vi "write_to_ini.vi"(7 "Enum":enum16{"Write", "Read variants", "Read Values"}(ring), 8 "error in (no error)":errorcluster, 9 "Input values":T1, 10 "String":string, 11 "configuration file path":path) -> (0 "error out":errorcluster, 1 "Output values":T1, 2 "section names":string[](array[string]), 3 "file path":path)   [LabVIEW 2021]
uses:
  <vilib>/Utility/config.llb/Write Key (String).vi
  <vilib>/Utility/config.llb/Read Key (String).vi
  <vilib>/Utility/config.llb/NI_LVConfig.lvlib
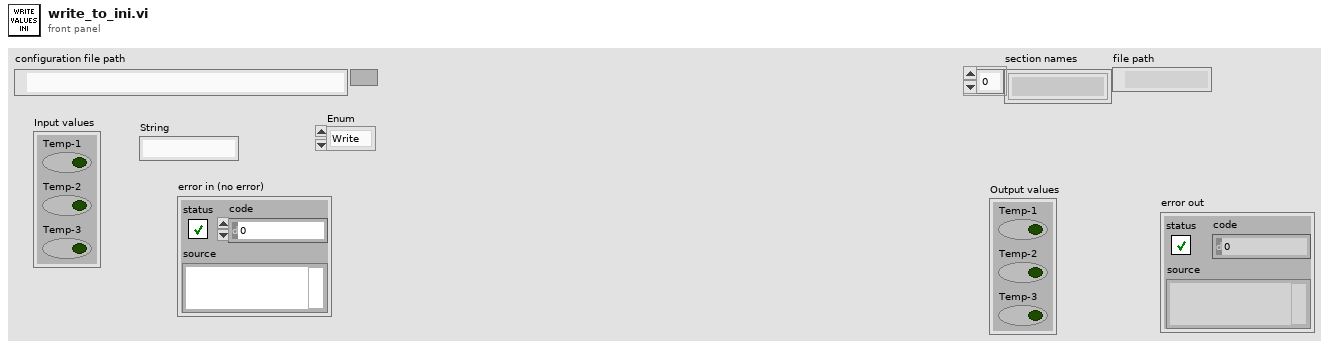
[diagram p1: front panel]
types:
  T1 = cluster{"Temp-1":bool, "Temp-2":bool, "Temp-3":bool}
  T2 = typedef "NI_LVConfig.lvlib/Config Data RefNum.ctl" = refnum<k1>
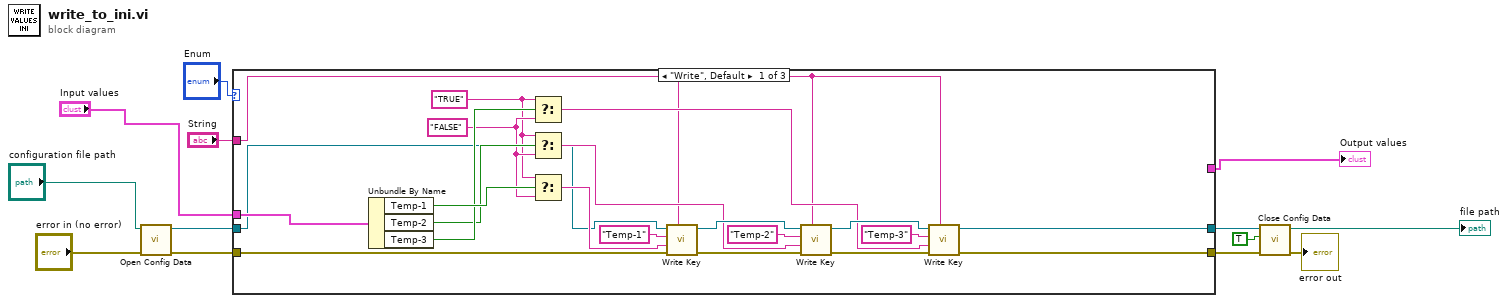
[diagram p0: block diagram]
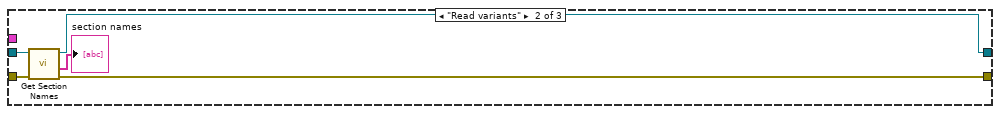
[diagram p2: hidden frame]
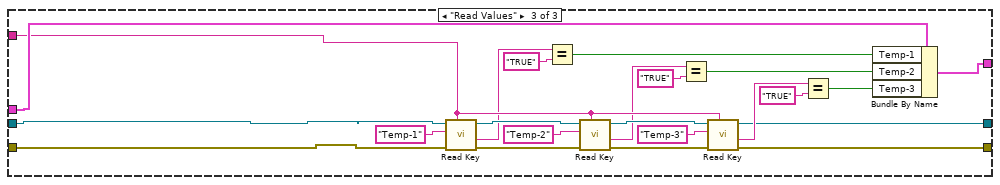
[diagram p3: hidden frame]
diagram:
  n1 = call <vilib>:"Open Config Data.vi"("error in (no error)"="error in (no error)", "configuration file path"="configuration file path") -> ("error out"=w9:errorcluster, "refnum"=w8:T2)  [unwired: 7 in, 1 out]
  n2 = case shown="\"Write\", Default" "Enum" {
    tunnel: w9 -> [w15 w35 w41]
    tunnel: w8 -> [w14 w36 w40]
    tunnel: "Input values" -> [w30 _ w62]
    tunnel: [w18 w38 w44] -> w5
    tunnel: [w17 w37 w43] -> w6
    tunnel: "String" -> [w16 _ w55]
    tunnel: [_ _ w42] -> w1
    frame "Write", Default {
      w26 = "FALSE"
      w25 = "TRUE"
      n3 = Unbundle By Name(w30) -> ("Temp-1"=w29:bool, "Temp-2"=w27:bool, "Temp-3"=w28:bool)
      n4 = Select(t=w25, s=w28, f=w26) -> (s? t:f=w22:string)
      n5 = Select(t=w25, s=w27, f=w26) -> (s? t:f=w23:string)
      n6 = Select(t=w25, s=w29, f=w26) -> (s? t:f=w24:string)
      n7 = call-poly <vilib>:"Write Key.vi"("section"=w16, "error in (no error)"=w15, "value"=w24, "key"="Temp-1", "refnum"=w14) -> ("error out"=w34:errorcluster, "refnum out"=w32:T2)  [unwired: 4 in, 1 out]
      n8 = call-poly <vilib>:"Write Key.vi"("section"=w16, "error in (no error)"=w34, "value"=w23, "key"="Temp-2", "refnum"=w32) -> ("error out"=w33:errorcluster, "refnum out"=w31:T2)  [unwired: 4 in, 1 out]
      n9 = call-poly <vilib>:"Write Key.vi"("section"=w16, "error in (no error)"=w33, "value"=w22, "key"="Temp-3", "refnum"=w31) -> ("error out"=w17:errorcluster, "refnum out"=w18:T2)  [unwired: 4 in, 1 out]
    }
    frame "Read variants" {
      n10 = call <vilib>:"Get Section Names.vi"("error in (no error)"=w35, "refnum"=w36) -> ("error out"=w37:errorcluster, "section names"=→"section names":string[], "refnum out"=w38:T2)  [unwired: 7 in]
    }
    frame "Read Values" {
      n11 = call-poly <vilib>:"Read Key.vi"("section"=w55, "error in (no error)"=w41, "key"="Temp-1", "refnum"=w40) -> ("error out"=w59:errorcluster, "value"=w52:string, "refnum out"=w60:T2)  [unwired: 4 in, 1 out]
      n12 = Equal?(x=w52, y="TRUE" ("key")) -> (x = y?=w45:bool)
      n13 = call-poly <vilib>:"Read Key.vi"("section"=w55, "error in (no error)"=w59, "key"="Temp-2", "refnum"=w60) -> ("error out"=w56:errorcluster, "value"=w50:string, "refnum out"=w57:T2)  [unwired: 4 in, 1 out]
      n14 = Equal?(x=w50, y="TRUE" ("key")) -> (x = y?=w46:bool)
      n15 = call-poly <vilib>:"Read Key.vi"("section"=w55, "error in (no error)"=w56, "key"="Temp-3", "refnum"=w57) -> ("error out"=w43:errorcluster, "value"=w48:string, "refnum out"=w44:T2)  [unwired: 4 in, 1 out]
      n16 = Equal?(x=w48, y="TRUE" ("key")) -> (x = y?=w47:bool)
      n17 = Bundle By Name(cluster=w62, "Temp-1"=w45, "Temp-2"=w46, "Temp-3"=w47) -> (w42:T1)
    }
  }
  "Output values" <- w1
  n18 = call <vilib>:"Close Config Data.vi"("error in (no error)"=w6, "write file if changed (T)"=TRUE, "refnum"=w5) -> ("error out"=→"error out":errorcluster, "file path"=→"file path":path)  [unwired: 7 in]
